vi "Is Available.vi"(8 "error in (no error)":errorcluster, 11 "Caraya Test Framework in":refnum<class "Caraya Test Framework.lvclass">) -> (0 "error out":errorcluster, 2 "Is Available":bool, 3 "Caraya Test Framework out":refnum<class "Caraya Test Framework.lvclass">)   [LabVIEW 2017, in "Framework.lvlib" / "Caraya Test Framework.lvclass"]
doc: "Indicates whether the test framework is currently available. This method must not directly link to the test framework."
uses:
  Caraya Test Framework.lvclass
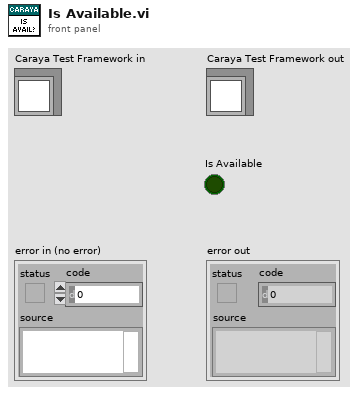
[diagram p1: front panel]
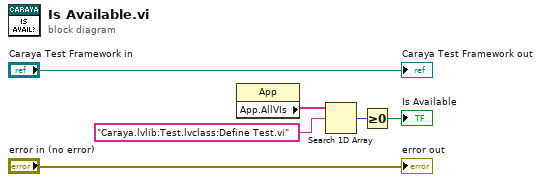
[diagram p0: block diagram]
diagram:
  n1 = property class="App"() -> ("App.AllVIs"=w4:string[])  [unwired: 2 in, 2 out]
  n2 = Search 1D Array(1D array=w4, element="Caraya.lvlib:Test.lvclass:Define Test.vi") -> (index of element=w2:i32)  [unwired: 1 in]
  n3 = Greater Or Equal To 0?(x=w2) -> (x >= 0?=→"Is Available":bool)
  "error out" <- "error in (no error)"
  "Caraya Test Framework out" <- "Caraya Test Framework in"
